vi "Process File.vi"(8 "error in (no error)":errorcluster, 10 "File":refnum<class "Acquired Result.lvclass">, 11 "Integrate in":refnum<class "Integrate.lvclass">) -> (0 "error out":errorcluster, 2 "File out":refnum<class "Acquired Result.lvclass">, 3 "Integrate out":refnum<class "Integrate.lvclass">)   [LabVIEW 2016, in "Integrate.lvclass"]
uses:
  Integrate.lvclass
  C:/Program Files/National Instruments/LabVIEW 2016/vi.lib/ActorFramework/Actor/Actor.lvclass
  NHMFL_Core/Libraries/Instruments/Results/Acquired Result/Acquired Result.lvclass
  <vilib>/ActorFramework/Actor/Actor.lvclass/Actor.ctl
  Channel peak.ctl
  LabActor Messages/Write Peak Field Msg/Write Peak Field Msg.lvclass/Write Peak Field Msg.ctl
  <vilib>/ActorFramework/Message Enqueuer/Message Enqueuer.lvclass/Message Enqueuer.ctl
  <vilib>/ActorFramework/Message Enqueuer/Enqueue.vi
  LabActor Messages/Write Peak Field Msg/Write Peak Field Msg.lvclass
  C:/Program Files/National Instruments/LabVIEW 2016/vi.lib/ActorFramework/Message/Message.lvclass
  Read Integrate Configuration.vi
  <vilib>/ActorFramework/Message Priority Queue/Priority Enqueue.vi
  <vilib>/ActorFramework/Actor/Actor.lvclass
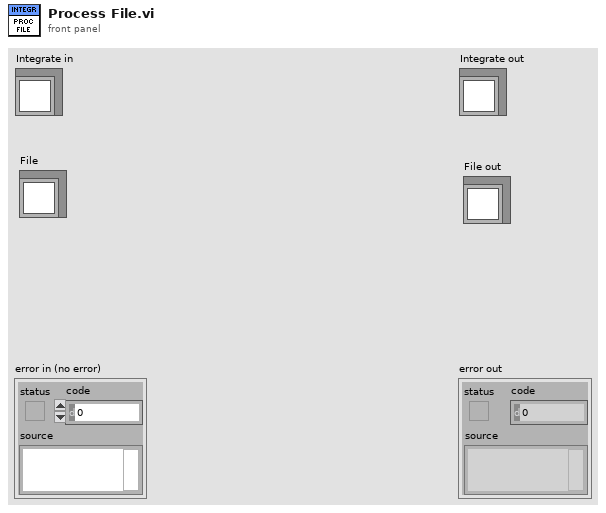
[diagram p1: front panel]
types:
  T1 = typedef "Integrator Configuration.ctl" = cluster{"Integrate":T2[], "Offset duration ":dbl, "TDMS group name":string}
  T2 = typedef "Integrate channel.ctl" = cluster{"Channel":string, "Output name":string, "Factor":dbl, "Start time":dbl, "Duration":dbl, "Fix drift":bool}
  T3 = typedef "Channel peak.ctl" = cluster{"Peak":dbl, "Name":string}
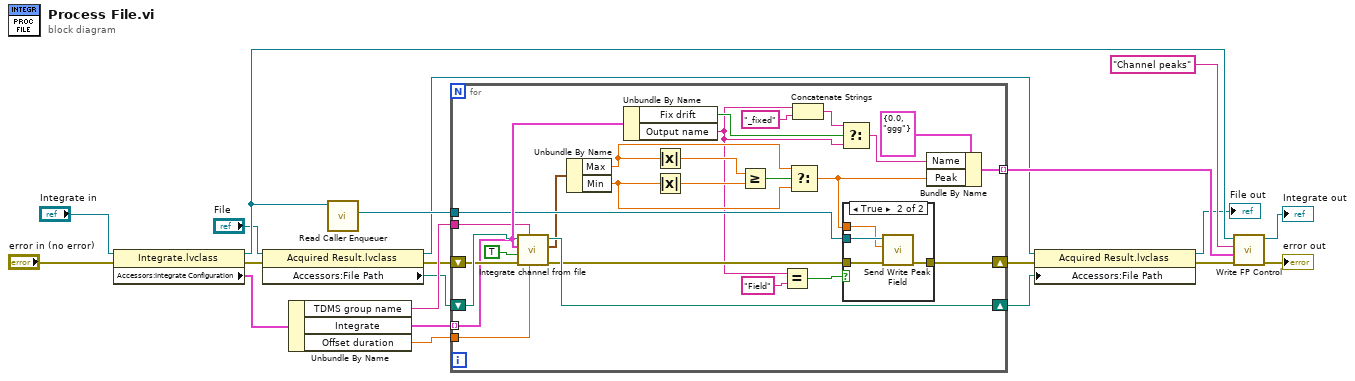
[diagram p0: block diagram]
diagram:
  n1 = property class="Integrate.lvclass"(reference="Integrate in", error in="error in (no error)") -> (reference out=w14:refnum<class "Integrate.lvclass">, error out=w4:errorcluster, "Accessors:Integrate Configuration"=w20:T1)
  n2 = property class="Acquired Result.lvclass"(reference="File", error in=w4) -> (reference out=w9:refnum<class "Acquired Result.lvclass">, error out=w3:errorcluster, "Accessors:File Path"=w7:path)
  n3 = Unbundle By Name(w20) -> ("TDMS group name"=w16:string, "Integrate"=w19:T2[], "Offset duration"=w18:dbl)
  n4 = call <vilib>:"Read Caller Enqueuer.vi"("Actor"=w14) -> ("Caller Enqueuer"=w17:refnum<class "Message Enqueuer.lvclass">)  [unwired: 10 in]
  n5 = for {
    tunnel: w19 -> [w42] mode=indexing
    shift-right: [w46] -> w5
    shift-left: w7 -> [w47]
    tunnel: w18 -> [w43]
    shift-right: [w38] -> w2
    shift-left: w3 -> [w44]
    tunnel: w17 -> [w37]
    tunnel: w16 -> [w36]
    tunnel: [w27] -> w11 mode=indexing
    n6 = call "Integrate channel from file.vi"("Offset duration"=w43, "group name"=w36, "Error In"=w44, "Save data"=TRUE, "Integration settings"=w42, "File Path Control"=w47) -> ("Error Out"=w39:errorcluster, "Min max"=w29:cluster{"Max":dbl, "Min":dbl}, "File Path out"=w46:path)  [unwired: 2 in, 1 out]
    n7 = Unbundle By Name(w29) -> ("Max"=w31:dbl, "Min"=w34:dbl)
    n8 = Unbundle By Name(w42) -> ("Fix drift"=w26:bool, "Output name"=w23:string)
    n9 = Absolute Value(x=w31) -> (abs(x)=w32:dbl)
    n10 = Absolute Value(x=w34) -> (abs(x)=w33:dbl)
    n11 = Greater Or Equal?(x=w32, y=w33) -> (x >= y?=w30:bool)
    n12 = Equal?(x=w23, y="Field") -> (x = y?=w40:bool)
    n13 = Select(t=w31, s=w30, f=w34) -> (s? t:f=w28:dbl)
    n14 = Concatenate Strings(w23, "_fixed" ("string")) -> (w22:string)
    n15 = Select(t=w22, s=w26, f=w23) -> (s? t:f=w25:string)
    n16 = case shown="True" w40 {
      tunnel: w39 -> [w48 w52]
      tunnel: [w48 w51] -> w38
      tunnel: w37 -> [_ w50]
      tunnel: w28 -> [_ w49]
      frame False {
      }
      frame True {
        n17 = call "Send Write Peak Field.vi"("error in (no error)"=w52, "Peak Field"=w49, "Message Enqueuer"=w50) -> ("error out"=w51:errorcluster)  [unwired: 7 in, 1 out]
      }
    }
    n18 = Bundle By Name(cluster=T3 {"Peak"=0.0, "Name"="ggg"} ("Channel peak"), "Name"=w25, "Peak"=w28) -> (w27:T3)
  }
  n19 = property class="Acquired Result.lvclass"(reference=w9, error in=w2, "Accessors:File Path"=w5) -> (reference out=→"File out":refnum<class "Acquired Result.lvclass">, error out=w1:errorcluster)
  n20 = call-dynamic "Write FP Control.vi"("error in (no error)"=w1, "Control Value"=w11, "Control Name"="Channel peaks", "Measure Object in"=w14) -> ("error out"=→"error out":errorcluster, "Measure Object out"=→"Integrate out":refnum<class "Integrate.lvclass">)  [unwired: 6 in]
